vi "Write RT FIFO.vi"(8 "error in":errorcluster, 11 "RT Data In":T1 {"Compiled Data"."9759 RevB"."Settings"."ControlCals"."ThetaLH (deg)" format="%.3f"; "Compiled Data"."9759 RevB"."Settings"."ControlCals"."ULHLag (sec)" format="%.3f"; "Compiled Data"."9759 RevB"."Settings"."ControlCals"."USLag (sec)" format="%.3f"; "Compiled Data"."9759 RevB"."Settings"."ControlCals"."TLead (sec)" format="%.3f"; "Compiled Data"."9759 RevB"."Settings"."ControlCals"."TLag (sec)" format="%.3f"}) -> (0 "error out":errorcluster, 3 "RT Data Out":T1 {"Compiled Data"."9759 RevB"."Settings"."ControlCals"."ThetaLH (deg)" format="%.3f"; "Compiled Data"."9759 RevB"."Settings"."ControlCals"."ULHLag (sec)" format="%.3f"; "Compiled Data"."9759 RevB"."Settings"."ControlCals"."USLag (sec)" format="%.3f"; "Compiled Data"."9759 RevB"."Settings"."ControlCals"."TLead (sec)" format="%.3f"; "Compiled Data"."9759 RevB"."Settings"."ControlCals"."TLag (sec)" format="%.3f"})   [LabVIEW 2015, in "NI 9759 RevB Custom Device.lvlib"]
uses:
  NI 9759 RevB Custom Device.lvlib
  Shared/Types/RT Data.ctl
  Shared/Types/Compiled Data.ctl
  Shared/Types/RT Init Data.ctl
  Shared/Types/RT Status.ctl
  Shared/Types/9759 RevB.ctl
  Shared/Types/FPGA Refs.ctl
  Shared/Types/Generic FPGA Ref.ctl
  Shared/Types/9759 RevB FPGA Ref.ctl
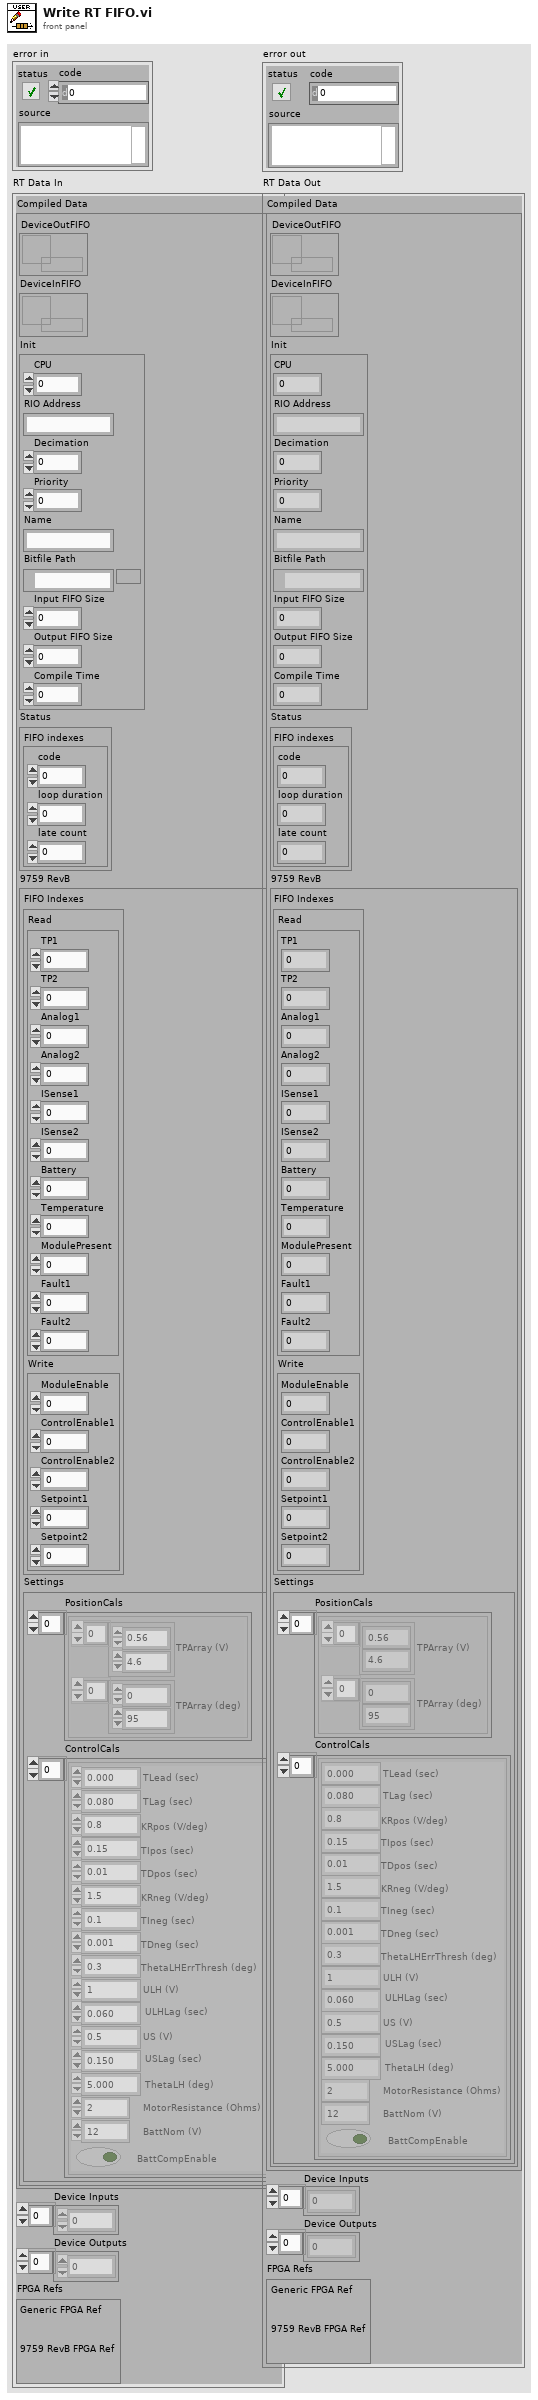
[diagram p1: front panel]
types:
  T1 = typedef "NI 9759 RevB Custom Device.lvlib/RT Data.ctl" = cluster{"Compiled Data":T2, "Device Inputs":dbl[], "Device Outputs":dbl[], "FPGA Refs":T6}
  T2 = typedef "NI 9759 RevB Custom Device.lvlib/Compiled Data.ctl" = cluster{"DeviceOutFIFO":refnum<k33>, "DeviceInFIFO":refnum<k33>, "Init":T3, "Status":T4, "9759 RevB":T5}
  T3 = typedef "NI 9759 RevB Custom Device.lvlib/RT Init Data.ctl" = cluster{"CPU":i32, "RIO Address":string, "Decimation":i32, "Priority":i32, "Name":string, "Bitfile Path":path, "Input FIFO Size":i32, "Output FIFO Size":i32, "Compile Time":dbl}
  T4 = typedef "NI 9759 RevB Custom Device.lvlib/RT Status.ctl" = cluster{"FIFO indexes":cluster{"code":i32, "loop duration":i32, "late count":i32}}
  T5 = typedef "NI 9759 RevB Custom Device.lvlib/9759 RevB.ctl" = cluster{"FIFO Indexes":cluster{"Read":cluster{"TP1":i32, "TP2":i32, "Analog1":i32, "Analog2":i32, "ISense1":i32, "ISense2":i32, "Battery":i32, "Temperature":i32, "ModulePresent":i32, "Fault1":i32, "Fault2":i32}, "Write":cluster{"ModuleEnable":i32, "ControlEnable1":i32, "ControlEnable2":i32, "Setpoint1":i32, "Setpoint2":i32}}, "Settings":cluster{"PositionCals":cluster{"TPArray (V)":sgl[], "TPArray (deg)":sgl[]}[], "ControlCals":cluster{"TLead (sec)":sgl, "TLag (sec)":sgl, "KRpos (V/deg)":sgl, "TIpos (sec)":sgl, "TDpos (sec)":sgl, "KRneg (V/deg)":sgl, "TIneg (sec)":sgl, "TDneg (sec)":sgl, "ThetaLHErrThresh (deg)":sgl, "ULH (V)":sgl, "ULHLag (sec)":sgl, "US (V)":sgl, "USLag (sec)":sgl, "ThetaLH (deg)":sgl, "MotorResistance (Ohms)":sgl, "BattNom (V)":sgl, "BattCompEnable":bool}[]}}
  T6 = typedef "NI 9759 RevB Custom Device.lvlib/FPGA Refs.ctl" = cluster{"Generic FPGA Ref":T7, "9759 RevB FPGA Ref":T8}
  T7 = typedef "NI 9759 RevB Custom Device.lvlib/Generic FPGA Ref.ctl" = refnum<k20>
  T8 = typedef "NI 9759 RevB Custom Device.lvlib/9759 RevB FPGA Ref.ctl" = refnum<k20>
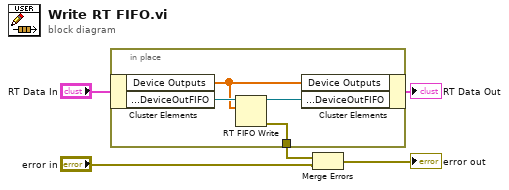
[diagram p0: block diagram]
diagram:
  n1 = in-place {
    in-place-border: [w6] -> w4
    n2 = in-place-cluster #1("RT Data In") -> ("Device Outputs"=w7:dbl[], "Compiled Data.DeviceOutFIFO"=w9:refnum<k33>)
    n3 = RT FIFO Write(0:w9, 1:w7) -> (8:w8:refnum<k33>, 11:w6:errorcluster)  [unwired: 3 in, 2 out]
    n4 = in-place-cluster #1("Device Outputs"=w7, "Compiled Data.DeviceOutFIFO"=w8) -> (→"RT Data Out":T1)
  }
  n5 = Merge Errors(w4, "error in") -> (→"error out":errorcluster)
